vi "ReadValues.vi"(8 "error in (no error)":errorcluster, 11 "Port":refnum<visa-resource-name>) -> (0 "error out":errorcluster, 1 "I":dbl, 2 "V":dbl, 3 "port out":refnum<visa-resource-name>, 4 "VIR":dbl[](array[numeric]))   [LabVIEW 2018]
uses:
  ThirdParty/Keithley 24XX/Keithley 24XX.lvlib
  ThirdParty/Keithley 24XX/Public/Data/Read (Measurements).vi
panel:
  out "R":dbl
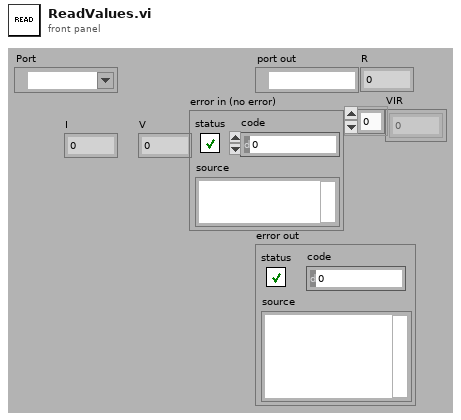
[diagram p1: front panel]
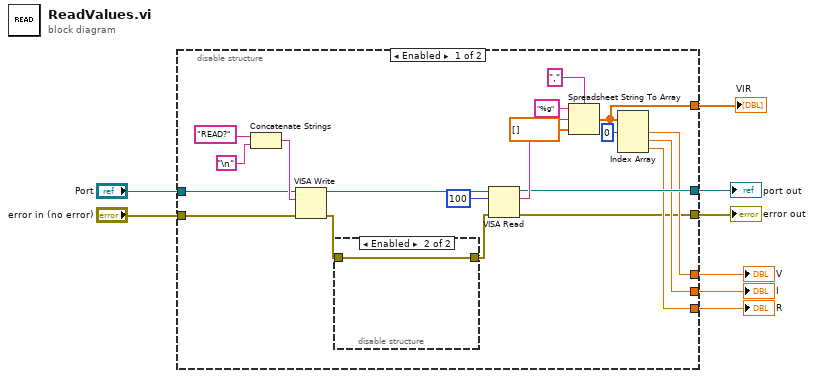
[diagram p0: block diagram]
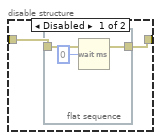
[diagram p2: hidden frame]
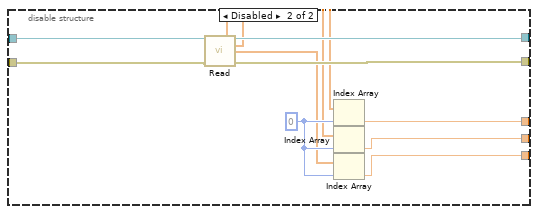
[diagram p3: hidden frame]
diagram:
  n1 = disable-structure shown="Enabled" {
    disable-tunnel: [w21 w41] -> w8
    disable-tunnel: "Port" -> [w19 w44]
    disable-tunnel: "error in (no error)" -> [w18 w43]
    disable-tunnel: [w11 w42] -> w5
    disable-tunnel: [w16 w36] -> w4
    disable-tunnel: [w14 w35] -> w3
    disable-tunnel: [w15 w34] -> w2
    disable-tunnel: [w9 _] -> w1
    frame Enabled {
      n2 = Concatenate Strings("READ?" ("data"), "\n") -> (w24:string)
      n3 = VISA Write(VISA resource name=w19, write buffer=w24, error in (no error)=w18) -> (VISA resource name out=w17:refnum<visa-resource-name>, error out=w13:errorcluster)  [unwired: 1 out]
      n4 = disable-structure shown="Enabled" {
        disable-tunnel: w13 -> [w30 w33]
        disable-tunnel: [w29 w33] -> w12
        frame Disabled {
          n5 = flat-sequence {
            tunnel: w30 -> [w31]
            tunnel: [w31] -> w29
            frame #0 {
              n6 = Wait (ms)(milliseconds to wait=u32 0) -> ()  [unwired: 1 out]
            }
          }
        }
        frame Enabled {
        }
      }
      n7 = VISA Read(VISA resource name=w17, byte count=100, error in (no error)=w12) -> (VISA resource name out=w21:refnum<visa-resource-name>, read buffer=w25:string, error out=w11:errorcluster)  [unwired: 1 out]
      n8 = Spreadsheet String To Array(delimiter (Tab)=",", format string="%g", spreadsheet string=w25, array type (2D Dbl)=dbl[] []) -> (array=w9:dbl[])
      n9 = Index Array(array=w9, index #1=0 ("index")) -> (element #1=w16:dbl, element #2=w14:dbl, element #3=w15:dbl)  [unwired: 2 in]
    }
    frame Disabled {
      w40 = 0 ("index")
      n10 = call-poly "Read.vi"("VISA resource name"=w44, "error in (no error)"=w43) -> ("Voltage Measurements"=w39:sgl[], "VISA resource name out"=w41:refnum<visa-resource-name>, "Current Measurements"=w38:sgl[], "Resistance Measurements"=w37:sgl[], "error out"=w42:errorcluster)  [unwired: 7 in, 2 out]
      n11 = Index Array(array=w39, index=w40) -> (element=w36:sgl)
      n12 = Index Array(array=w38, index=w40) -> (element=w35:sgl)
      n13 = Index Array(array=w37, index=w40) -> (element=w34:sgl)
    }
  }
  "V" <- w4
  "I" <- w3
  "port out" <- w8
  "error out" <- w5
  "R" <- w2
  "VIR" <- w1
